vi "air flow calibrator (source sensor).vi"(4 "State":i16, 5 "Time":dbl format="%.2f", 6 "Sensor Values":dbl[](array[numeric])=[120000.0, 10000.0], 7 "Set Points":dbl[](array[numeric])=[1.0, 22.0, 5e-05]) -> (0 "required data":T1={"Set Point names"=["accumulator volume (L)", "air temperature (C)", "calibration state number"], "required number of setpoints"=3, "required number of sensors"=2, "Sensor names"=["Accumulator pressure (Pa)", "Source pressure (Pa)"]}, 3 "output value":dbl)   [LabVIEW 2015]
uses:
  <vilib>/Analysis/NI_AALPro.lvlib
panel:
  # "Enter the correct information for this control code in the required data structure below. Then make the current value default by right clicking on the border of the data structure."
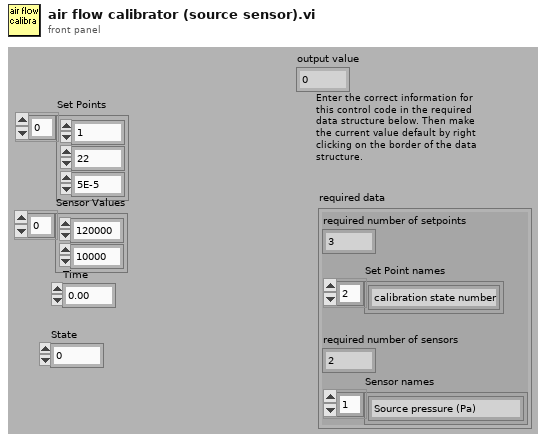
[diagram p1: front panel]
types:
  T1 = cluster{"Set Point names":string[], "required number of setpoints":u8, "required number of sensors":u8, "Sensor names":string[]}
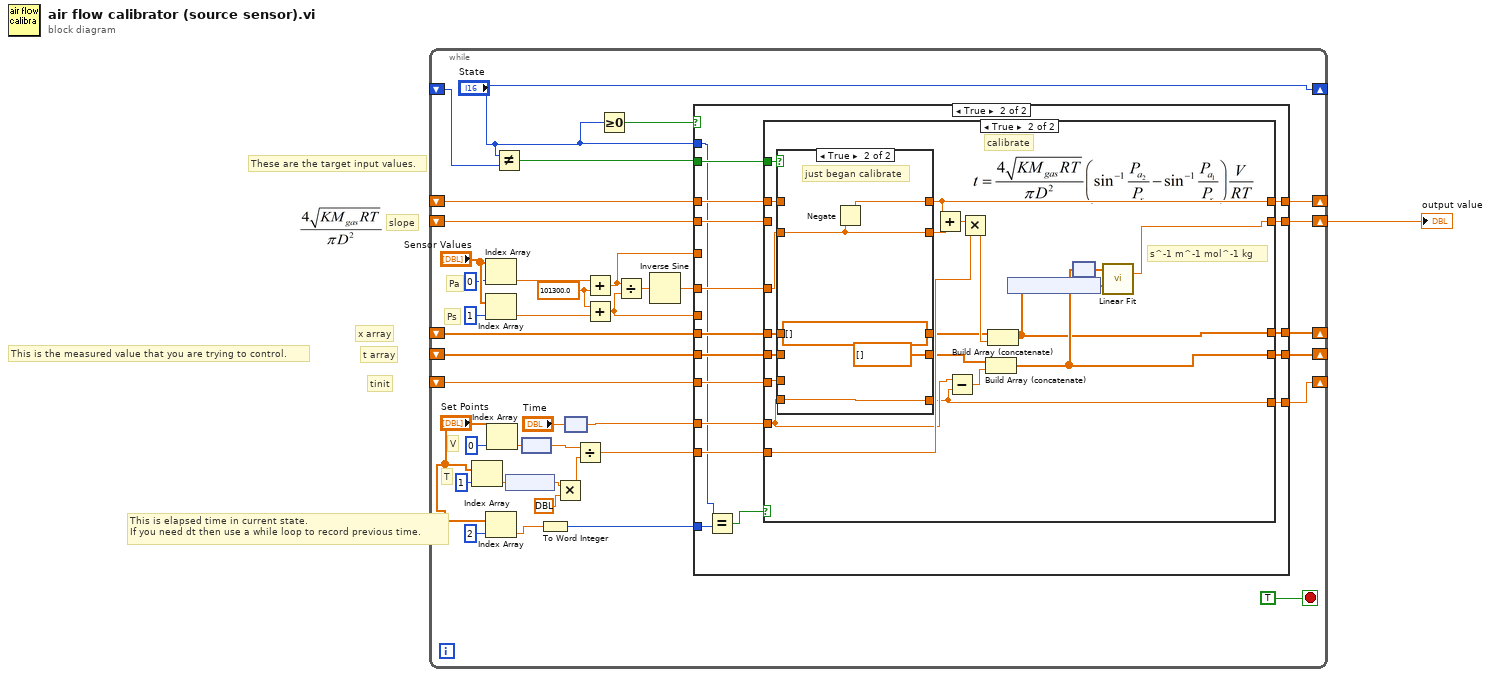
[diagram p0: block diagram]
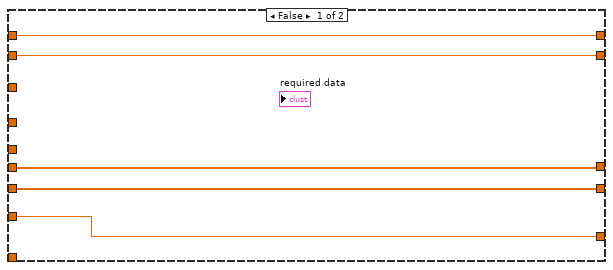
[diagram p2: hidden frame]
diagram:
  # "slope"
  # "tinit"
  # "t array"
  # "x array"
  # "These are the target input values."
  # "This is the measured value that you are trying to control."
  # "This is elapsed time in current state.\nIf you need dt then use a while loop to record previous time."
  n1 = while {
    shift-right: ["State"] -> _
    shift-left: _ -> [w4]
    shift-right: [w37] -> _
    shift-left: _ -> [w36]
    shift-right: [w23] -> _
    shift-left: _ -> [w24]
    shift-right: [w21] -> _
    shift-left: _ -> [w22]
    shift-right: [w19] -> _
    shift-left: _ -> [w18]
    shift-right: [w17] -> w1
    shift-left: _ -> [w16]
    stop <- TRUE stop-if-true
    w9 = 101300.0 ("y")
    # "T"
    # "V"
    # "Ps"
    # "Pa"
    n2 = Index Array(array="Set Points", index=1) -> (element=w31:dbl)
    n3 = Index Array(array="Sensor Values", index=0) -> (element=w13:dbl)
    n4 = Index Array(array="Sensor Values", index=1) -> (element=w12:dbl)
    n5 = Index Array(array="Set Points", index=2) -> (element=w6:dbl)
    n6 = Index Array(array="Set Points", index=0) -> (element=w32:dbl)
    n7 = Not Equal?(x="State", y=w4) -> (x != y?=w38:bool)
    n8 = node(w31) -> (w29:dbl[unit])
    n9 = node(w32) -> (w30:dbl[unit])
    n10 = To Word Integer(number=w6) -> (16bit integer=w5:i16)
    n11 = Multiply(x=w29, y=ext[unit] 8.314472) -> (x*y=w27:ext[unit])
    n12 = node("Time") -> (w20:dbl[unit])
    n13 = Divide(x=w30, y=w27) -> (x/y=w26:ext[unit])
    n14 = Add(x=w13, y=w9) -> (x+y=w10:dbl)
    n15 = Add(x=w9, y=w12) -> (x+y=w11:dbl)
    n16 = Greater Or Equal To 0?(x="State") -> (x >= 0?=w3:bool)
    n17 = Divide(x=w10, y=w11) -> (x/y=w35:dbl)
    n18 = Inverse Sine(1:w35) -> (0:w34:dbl)
    n19 = case shown="True" w3 {
      tunnel: w38 -> [_ w63]
      tunnel: w34 -> [_ w62]
      tunnel: [w45 w60] -> w37
      tunnel: w36 -> [w45 w61]
      tunnel: w26 -> [_ w59]
      tunnel: w20 -> [_ w53]
      tunnel: w24 -> [w44 w58]
      tunnel: [w44 w55] -> w23
      tunnel: w22 -> [w43 w57]
      tunnel: [w43 w56] -> w21
      tunnel: [w42 w52] -> w19
      tunnel: w18 -> [w42 w54]
      tunnel: [w46 w51] -> w17
      tunnel: w16 -> [w46 w48]
      tunnel: w10 -> [_ _]
      tunnel: w11 -> [_ _]
      tunnel: w5 -> [_ w50]
      tunnel: "State" -> [_ w47]
      frame False {
      }
      frame True {
        n20 = Equal?(x=w47, y=w50) -> (x = y?=w49:bool)
        n21 = case shown="True" w49 {
          tunnel: w63 -> [_ w89]
          tunnel: w62 -> [_ w88]
          tunnel: w61 -> [w68 w87]
          tunnel: [w68 w86] -> w60
          tunnel: w59 -> [_ w84]
          tunnel: w58 -> [w66 w80]
          tunnel: w57 -> [w65 w78]
          tunnel: [w65 w77] -> w56
          tunnel: [w66 w76] -> w55
          tunnel: w54 -> [w64 w75]
          tunnel: w53 -> [_ w74]
          tunnel: [w64 w73] -> w52
          tunnel: [w67 w69] -> w51
          tunnel: w48 -> [w67 _]
          frame False {
          }
          frame True {
            # "s^-1 m^-1 mol^-1 kg"
            # "calibrate"
            n22 = case shown="True" w89 {
              tunnel: w88 -> [w93 w98]
              tunnel: [w94 w99] -> w86
              tunnel: w87 -> [w94 _]
              tunnel: [w93 w98] -> w83
              tunnel: [w92 ext[unit][] []] -> w81
              tunnel: w80 -> [w92 _]
              tunnel: [w91 dbl[unit][] []] -> w79
              tunnel: w78 -> [w91 _]
              tunnel: [w90 w95] -> w73
              tunnel: w74 -> [_ w95]
              tunnel: w75 -> [w90 _]
              frame False {
              }
              frame True {
                # "just began calibrate"
                n23 = Negate(x=w98) -> (-x=w99:dbl)
              }
            }
            n24 = Add(x=w86, y=w83) -> (x+y=w85:dbl)
            n25 = Subtract(x=w74, y=w73) -> (x-y=w72:dbl[unit])
            n26 = Multiply(x=w85, y=w84) -> (x*y=w82:ext[unit])
            n27 = Build Array (concatenate)(w79, w72) -> (w77:dbl[unit][])
            n28 = Build Array (concatenate)(w81, w82) -> (w76:ext[unit][])
            n29 = node(w76) -> (w70:ext[])
            n30 = node(w77) -> (w71:dbl[])
            n31 = call <vilib>:"Linear Fit.vi"("Y"=w71, "X"=w70) -> ("slope"=w69:dbl)  [unwired: 9 in, 4 out]
          }
        }
      }
    }
  }
  "output value" <- w1
